vi "AOL Z Cal-Wizard window.vi"(8 "error in (no error)":errorcluster) -> (0 "error out":errorcluster, 1 "Cancelled":bool)   [LabVIEW 2013]
doc: "Use this template to create a dialog box with event handling."
uses:
  Typedefs/Cal points.ctl
  Typedefs/Cal mode.ctl
  Typedefs/Cal channel.ctl
  Typedefs/Pre-AOL Z wizard refs.ctl
  <vilib>/Utility/miscctls.llb/LVPointTypeDef.ctl
  Typedefs/AOL Z cal wizard states.ctl
  Global Variables/General Globals.vi
  Globals/gl_Calibration globals.vi
panel:
  out "Message":string
  out "Note":string
  in  "Channel Selector":T1
  in  "Calibration Mode":T2
  in  "Cal points":T3=enum."21-points calibration" caption="Select desired number of calibration points"
  in  "Back":bool
  in  "Next":bool
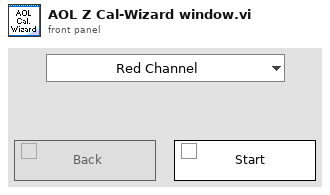
[diagram p1: front panel]
types:
  T1 = typedef "Cal channel.ctl" = enum16{"Red Channel", "Green Channel"}
  T2 = typedef "Cal mode.ctl" = enum16{"Automatic", "Interactive"}
  T3 = typedef "Cal points.ctl" = enum16{"5-points calibration (crude)", "11-points calibration", "21-points calibration", "41-points calibration"}
  T4 = typedef "Pre-AOL Z wizard refs.ctl" = cluster{"VI's reference":refnum<vi>, "Calibration Mode":refnum<vi>, "Cal points":refnum<vi>, "Channel Selector":refnum<vi>, "Message":refnum<vi>, "Back":refnum<vi>, "Next":refnum<vi>, "Power meter AI":refnum<vi>, "2D Picture":refnum<vi>, "Note":refnum<vi>}
  T5 = typedef "AOL Z cal wizard states.ctl" = enum16{"Idle", "Select cal mode", "Select cal points", "Select channel", "Start calibration"}
  T6 = typedef "LVPointTypeDef.ctl" = cluster{"Horizontal":i16, "Vertical":i16}
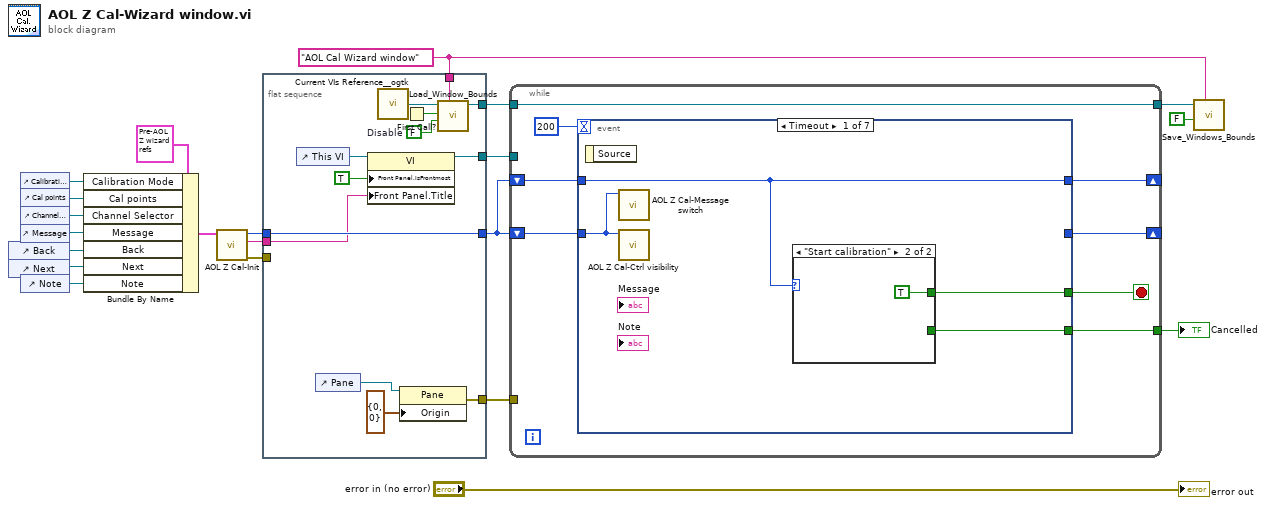
[diagram p0: block diagram]
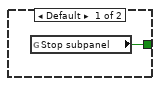
[diagram p2: hidden frame]
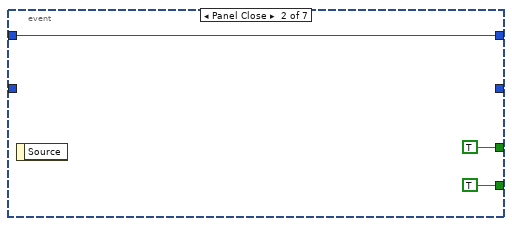
[diagram p3: hidden frame]
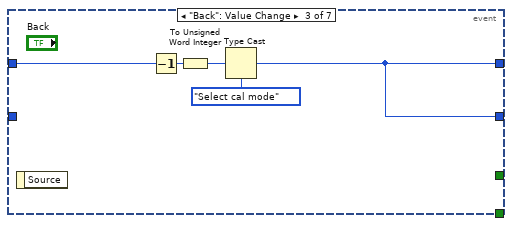
[diagram p4: hidden frame]
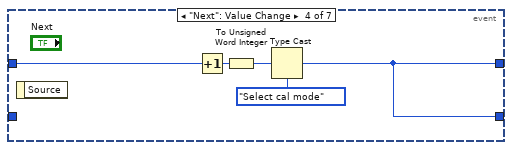
[diagram p5: hidden frame]
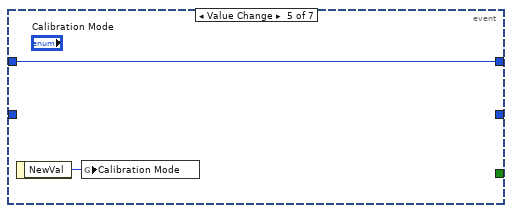
[diagram p6: hidden frame]
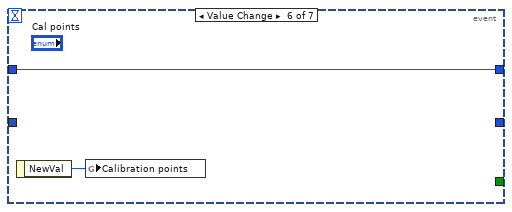
[diagram p7: hidden frame]
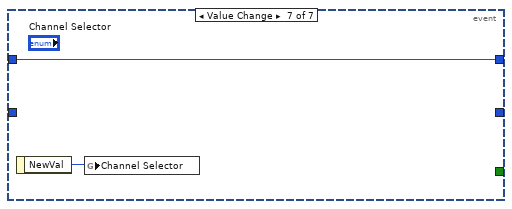
[diagram p8: hidden frame]
diagram:
  w9 = "AOL Cal Wizard window" ("Window Name (i.e. Key)")
  n1 = control-ref of="Back"() -> (w7:refnum<vi>)
  n2 = control-ref of="Next"() -> (w6:refnum<vi>)
  n3 = control-ref of="Calibration Mode"() -> (w12:refnum<vi>)
  n4 = control-ref of="Cal points"() -> (w13:refnum<vi>)
  n5 = control-ref of="Channel Selector"() -> (w14:refnum<vi>)
  n6 = control-ref of="Message"() -> (w2:refnum<vi>)
  n7 = control-ref of="Note"() -> (w1:refnum<vi>)
  n8 = Bundle By Name(cluster=T4 {"VI's reference"=refnum, "Calibration Mode"=refnum, "Cal points"=refnum, "Channel Selector"=refnum, "Message"=refnum, "Back"=refnum, "Next"=refnum, "Power meter AI"=refnum, "2D Picture"=refnum, "Note"=refnum} ("Pre-AOL Z wizard refs"), "Calibration Mode"=w12, "Cal points"=w13, "Channel Selector"=w14, "Message"=w2, "Back"=w7, "Next"=w6, "Note"=w1) -> (w10:T4)
  n9 = call "AOL Z Cal-Init.vi"("Pre-AOL Z wizard refs"=w10) -> ("error out"=w8:errorcluster, "Cal settings window's title"=w3:string, "Initial state"=w4:T5)  [unwired: 8 in]
  n10 = flat-sequence {
    tunnel: [w32] -> w21
    tunnel: [w30] -> w20
    tunnel: [w25] -> w18
    tunnel: [w23] -> w5
    tunnel: w9 -> [w24]
    tunnel: w8 -> [_]
    tunnel: w4 -> [w23]
    tunnel: w3 -> [w22]
    frame #0 {
      w26 = FALSE  # Disable
      n11 = control-ref of="This VI"() -> (w33:refnum<vi>)
      n12 = control-ref of="Pane"() -> (w29:refnum<vi>)
      n13 = property on="Property Node" class="VI"(reference=w33, "Front Panel.IsFrontmost"=TRUE ("Front Panel Window:Is Frontmost"), "Front Panel.Title"=w22) -> (reference out=w32:refnum<vi>)  [unwired: 1 in, 1 out]
      n14 = call "Current VIs Reference__ogtk.vi"() -> ("Current VI's reference"=w28:refnum<vi>)  [unwired: 5 in]
      n15 = property class="Pane"(reference=w29, "Origin"=T6 {"Horizontal"=0, "Vertical"=0}) -> (error out=w30:errorcluster)  [unwired: 1 in, 1 out]
      n16 = First Call?() -> (First Call?: T/F=w27:bool)
      n17 = call "Load_Window_Bounds.vi"("Window Name (i.e. Key)"=w24, "Disable"=w26, "First Call"=w27, "Window VI's Ref"=w28) -> ("reference out"=w25:refnum<vi>)  [unwired: 4 in, 3 out]
    }
  }
  n18 = while {
    tunnel: w20 -> [_]
    tunnel: w21 -> [_]
    tunnel: [w40] -> w15
    tunnel: w18 -> [w39]
    tunnel: [w39] -> w17
    shift-right: [w35] -> _
    shift-left: w5 -> [w38]
    shift-right: [w37] -> _
    shift-left: w5 -> [w36]
    stop <- w42 stop-if-true
    n19 = event shown="[0] Timeout" {
      selector: _ -> [_ _ _ _ _ _ _]
      dyn-events: _ -> [_ _ _ _ _ _ _]
      timeout: 200 -> [_ _ _ _ _ _ _]
      tunnel: [w44 TRUE ("Stop?") _ _ _ _ _] -> w42
      tunnel: [w43 TRUE ("Stop subpanel") _ _ _ _ _] -> w40
      tunnel: w38 -> [w46 _ _ _ _ _ _]
      tunnel: [w45 w49 w52 w60 w62 w64 w66] -> w37
      tunnel: w36 -> [w45 w49 w53 w61 w62 w64 w66]
      tunnel: [_ _ w52 w60 _ _ _] -> w35
      event Timeout {
        n20 = event-data() -> ()  [unwired: 1 in, 1 out]
        n21 = call "AOL Z Cal-Message switch.vi"("State"=w46) -> ()  [unwired: 10 in, 1 out]
        n22 = call "AOL Z Cal-Ctrl visibility.vi"("State"=w46) -> ()  [unwired: 10 in, 1 out]
        n23 = case shown="\"Start calibration\"" w45 {
          tunnel: [_ TRUE] -> w44
          tunnel: [w47 _] -> w43
          frame Default {
            n24 = global read "General Globals.vi" "Stop subpanel"() -> (w47:bool)
          }
          frame "Start calibration" {
          }
        }
      }
      event Panel Close {
        n25 = event-data() -> ()  [unwired: 1 in, 1 out]
      }
      event "Back": Value Change {
        n26 = event-data() -> ()  [unwired: 1 in, 1 out]
        n27 = Decrement(x=w53) -> (x-1=w54:T5)
        n28 = To Unsigned Word Integer(number=w54) -> (unsigned 16bit integer=w55:u16)
        n29 = Type Cast(type=AOL_Z_cal_wizard_states."Select cal mode" ("States"), x=w55) -> (*(type *) &x=w52:T5)
      }
      event "Next": Value Change {
        n30 = event-data() -> ()  [unwired: 1 in, 1 out]
        n31 = Increment(x=w61) -> (x+1=w57:T5)
        n32 = To Unsigned Word Integer(number=w57) -> (unsigned 16bit integer=w58:u16)
        n33 = Type Cast(type=AOL_Z_cal_wizard_states."Select cal mode" ("States"), x=w58) -> (*(type *) &x=w60:T5)
      }
      event Value Change {
        n34 = event-data() -> ("NewVal"=w63:T2)  [unwired: 1 in]
        n35 = global write "gl_Calibration globals.vi" "Calibration Mode"(w63) -> ()
      }
      event Value Change {
        n36 = event-data() -> ("NewVal"=w65:T3)  [unwired: 1 in]
        n37 = global write "gl_Calibration globals.vi" "Calibration points"(w65) -> ()
      }
      event Value Change {
        n38 = event-data() -> ("NewVal"=w67:T1)  [unwired: 1 in]
        n39 = global write "gl_Calibration globals.vi" "Channel Selector"(w67) -> ()
      }
    }
  }
  "Cancelled" <- w15
  n40 = call "Save_Windows_Bounds.vi"("Window Name (i.e. Key)"=w9, "Front Panel Window:Open"=FALSE, "Window VI's Ref"=w17) -> ()  [unwired: 8 in, 1 out]
  "error out" <- "error in (no error)"
